vi "Connect Error Terminals.vi"(8 "error in (no error)":errorcluster, 11 "VI Path":path) -> (0 "error out":errorcluster)   [LabVIEW 2016, in "SLL Class DVR API Generator.lvlib"]
uses:
  SLL Class DVR API Generator.lvlib
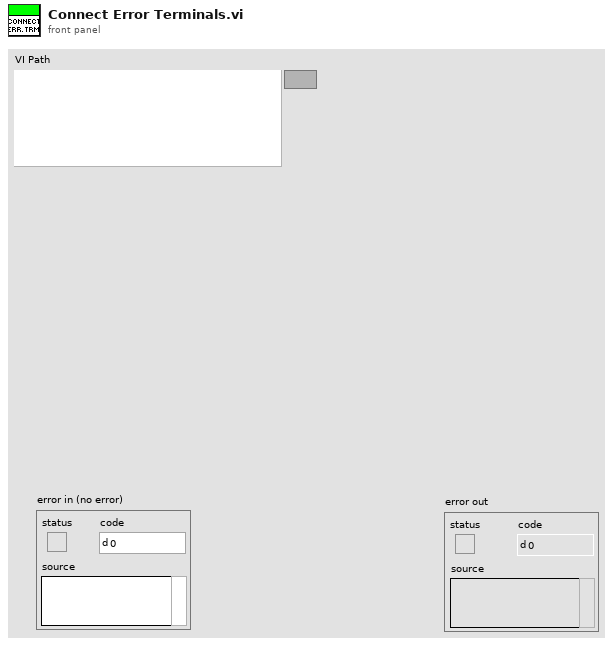
[diagram p1: front panel]
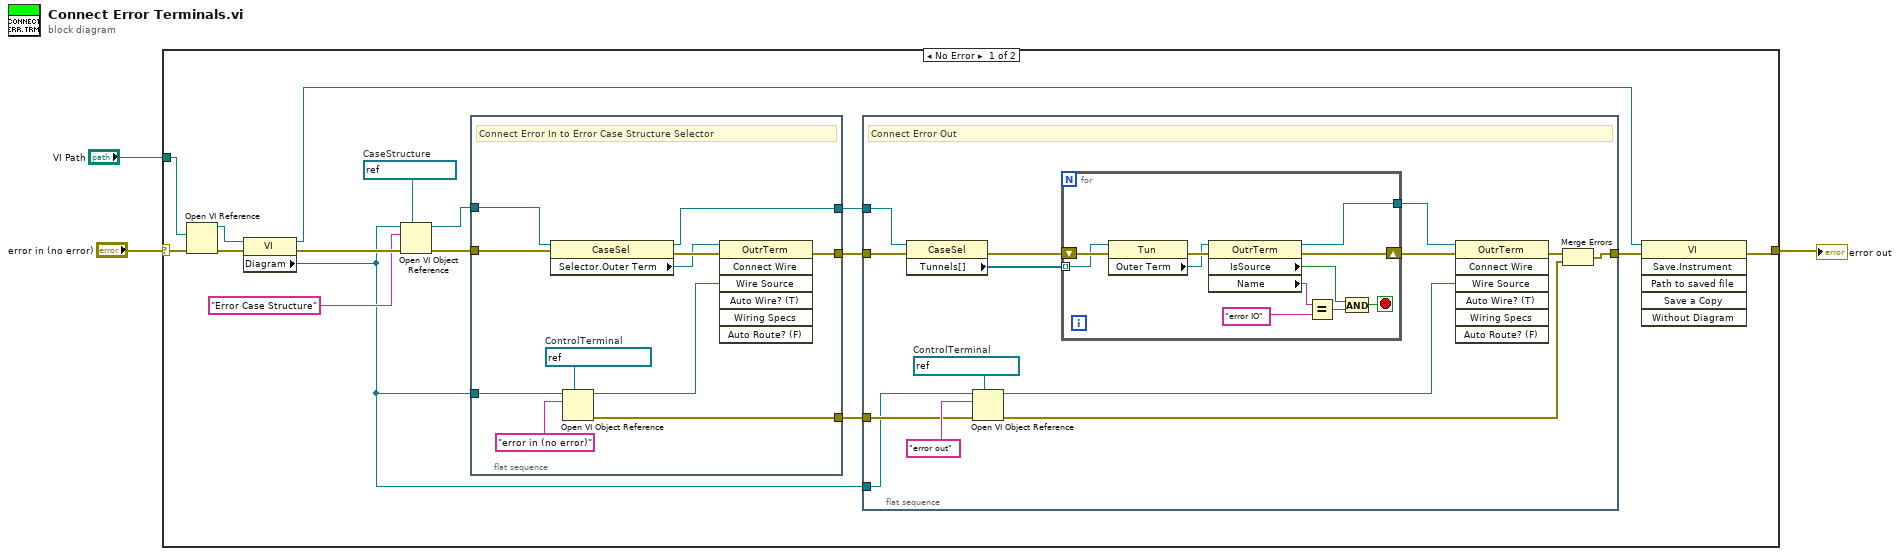
[diagram p0: block diagram]
diagram:
  n1 = case shown="No Error" "error in (no error)" {
    selector: "error in (no error)" -> [w19 w56]
    tunnel: [w5 w56] -> w2
    tunnel: "VI Path" -> [w17 _]
    frame No Error {
      w13 = refnum<vi> refnum  # CaseStructure
      n2 = Open VI Reference(vi path=w17, error in (no error)=w19) -> (vi reference=w15:refnum<vi>, error out=w18:errorcluster)  [unwired: 4 in]
      n3 = property class="VI"(reference=w15, error in=w18) -> (reference out=w4:refnum<vi>, error out=w16:errorcluster, "Diagram"=w6:refnum<vi>)
      n4 = Open VI Object Reference(7:w13, 8:w16, 10:"Error Case Structure" ("name/order"), 11:w6) -> (0:w12:errorcluster, 3:w11:refnum<vi>)
      n5 = flat-sequence {
        tunnel: w6 -> [w55]
        tunnel: w12 -> [w52]
        tunnel: w11 -> [w50]
        tunnel: [w49] -> w10
        tunnel: [w46] -> w8
        tunnel: [w45] -> w7
        frame #0 {
          w53 = refnum<vi> refnum  # ControlTerminal
          # "Connect Error In to Error Case Structure Selector"
          n6 = property class="CaseSel"(reference=w50, error in=w52) -> (reference out=w46:refnum<vi>, error out=w51:errorcluster, "Selector.Outer Term"=w48:refnum<vi>)
          n7 = Open VI Object Reference(7:w53, 10:"error in (no error)" ("name/order"), 11:w55) -> (0:w45:errorcluster, 3:w47:refnum<vi>)  [unwired: 1 in]
          n8 = invoke class="OutrTerm" method="Connect Wire"(reference=w48, error in=w51, "Wire Source"=w47) -> (error out=w49:errorcluster)  [unwired: 4 in, 6 out]
        }
      }
      n9 = flat-sequence {
        tunnel: w10 -> [w33]
        tunnel: [w21] -> w9
        tunnel: w8 -> [w31]
        tunnel: w7 -> [w26]
        tunnel: w6 -> [w25]
        frame #0 {
          w28 = refnum<vi> refnum  # ControlTerminal
          # "Connect Error Out"
          n10 = property class="CaseSel"(reference=w31, error in=w33) -> (error out=w32:errorcluster, "Tunnels[]"=w29:refnum<vi>[])  [unwired: 1 out]
          n11 = Open VI Object Reference(7:w28, 8:w26, 10:"error out" ("name/order"), 11:w25) -> (0:w20:errorcluster, 3:w22:refnum<vi>)
          n12 = for {
            shift-right: [w36] -> w30
            shift-left: w32 -> [w44]
            tunnel: w29 -> [w43] mode=indexing
            tunnel: [w34] -> w23
            stop <- w35 stop-if-true
            n13 = property class="Tun"(reference=w43, error in=w44) -> (error out=w42:errorcluster, "Outer Term"=w41:refnum<vi>)  [unwired: 1 out]
            n14 = property class="OutrTerm"(reference=w41, error in=w42) -> (reference out=w34:refnum<vi>, error out=w36:errorcluster, "IsSource"=w37:bool, "Name"=w40:string)
            n15 = Equal?(x=w40, y="error IO") -> (x = y?=w38:bool)
            n16 = And(x=w37, y=w38) -> (x .and. y?=w35:bool)
          }
          n17 = invoke class="OutrTerm" method="Connect Wire"(reference=w23, error in=w30, "Wire Source"=w22) -> (error out=w24:errorcluster)  [unwired: 4 in, 6 out]
          n18 = Merge Errors(w24, w20) -> (w21:errorcluster)
        }
      }
      n19 = invoke class="VI" method="Save.Instrument"(reference=w4, error in=w9) -> (error out=w5:errorcluster)  [unwired: 4 in, 5 out]
    }
    frame Error {
    }
  }
  "error out" <- w2
